vi "PreparePassReceiverRole.vi"(5 "Striker/2ndStriker":T1, 6 "Tactic index in":i32, 7 "first call":bool, 8 "error in (no error)":errorcluster, 9 "RobotRef":refnum<class "Robot.lvclass">, 10 "Game in":refnum<class "Game.lvclass">, 11 "PreparePassReceiverRole in":refnum<class "PreparePassReceiverRole.lvclass">) -> (0 "error out":errorcluster, 1 "Robot out":refnum<class "Robot.lvclass">, 2 "Game out":refnum<class "Game.lvclass">, 3 "PreparePassReceiverRole out":refnum<class "PreparePassReceiverRole.lvclass">, 4 "tactic index":i32)   [LabVIEW 2023, in "PreparePassReceiverRole.lvclass"]
uses:
  PreparePassReceiverRole.lvclass
  Game_class/Game.lvclass
  Robot_class/Robot.lvclass
  PreparePassReceiverEnum.ctl
  Role_class/Role.lvclass/Role.ctl
  PositionToReceivePassTactic_class/PositionToReceivePassTactic.lvclass/PositionToReceivePassTactic.ctl
  PositionToReceivePassTactic_class/Read States.vi
  Role_class/Read Tacticbook.vi
  Role_class/Write Tacticbook.vi
  Role_class/Write tactic_index.vi
  Tacticbook_class/Tacticbook.lvclass
  PositionToReceivePassTactic_class/PositionToReceivePassTactic.lvclass
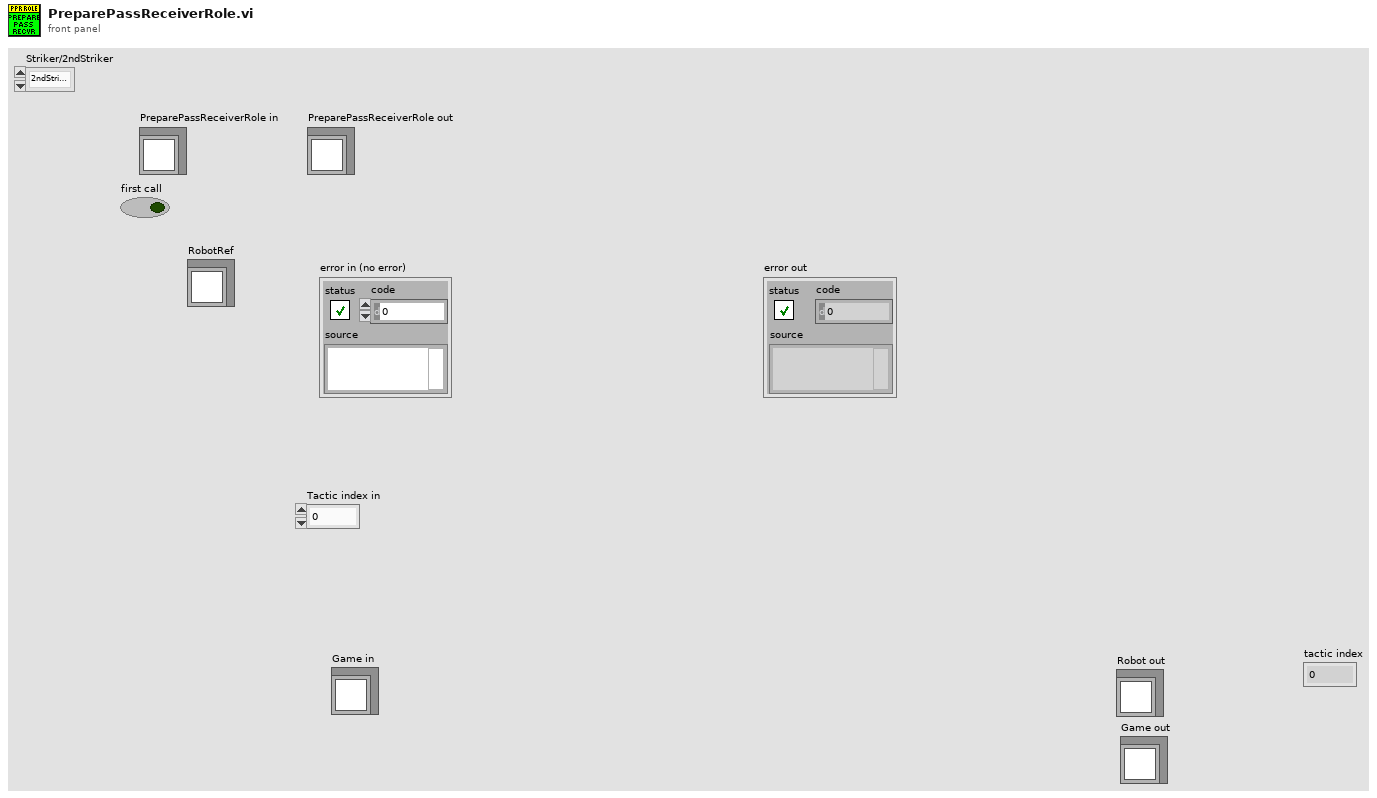
[diagram p1: front panel]
types:
  T1 = typedef "PreparePassReceiverEnum.ctl" = enum16{"2ndStrikerDPass", "2ndStriker", "Striker"}
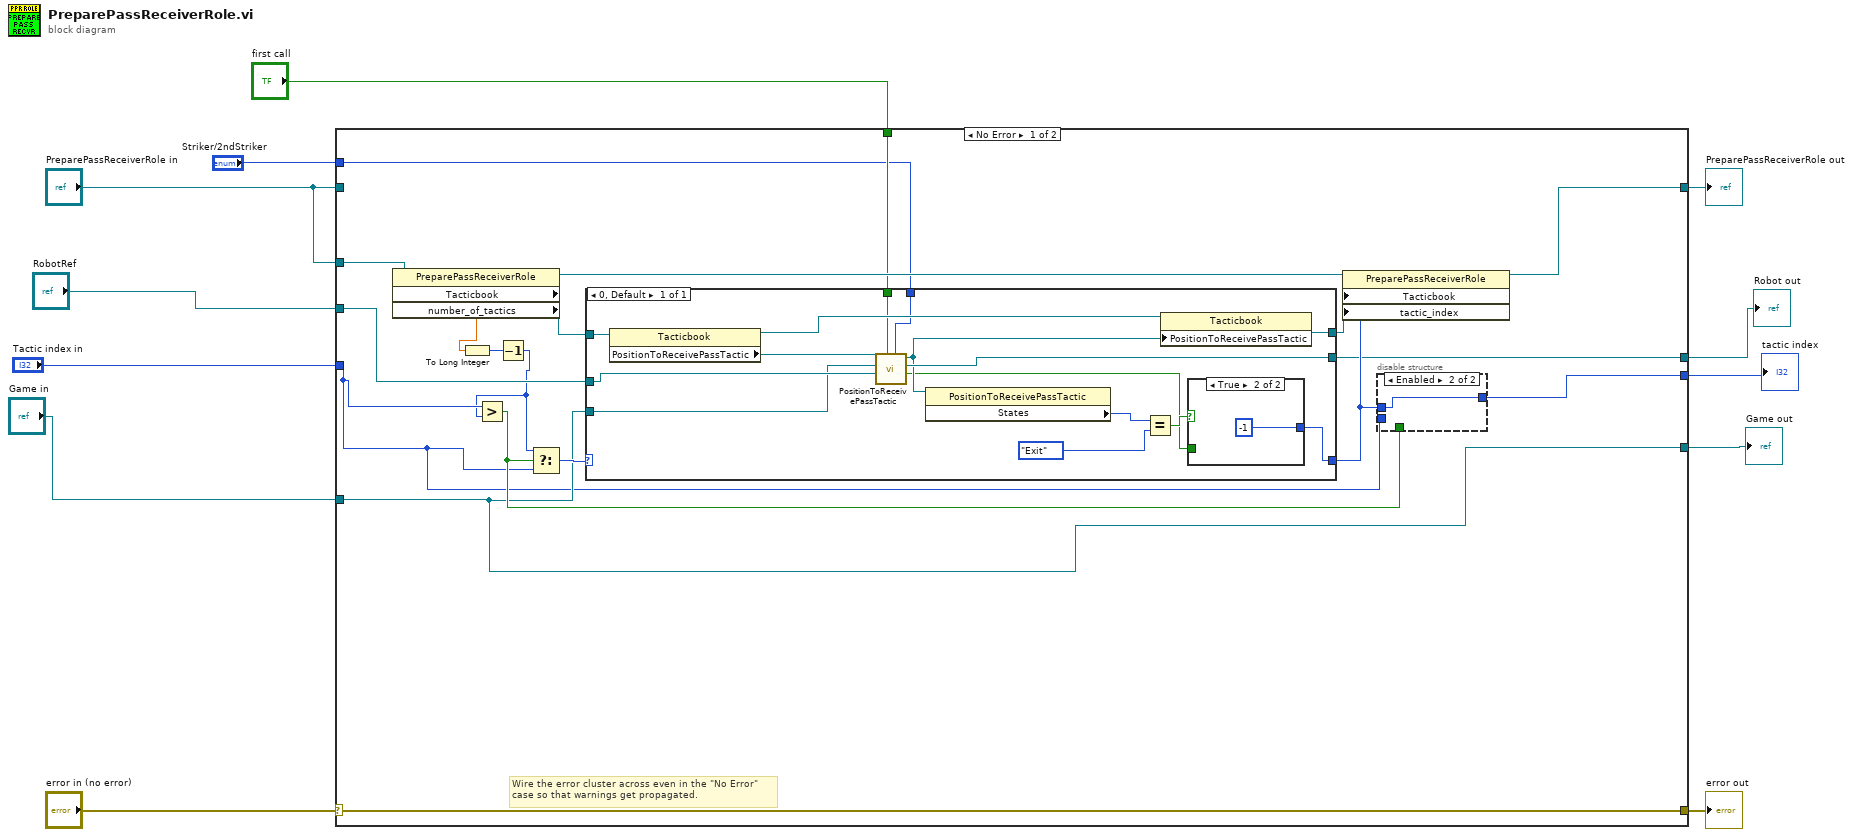
[diagram p0: block diagram]
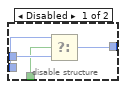
[diagram p2: hidden frame]
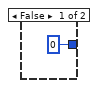
[diagram p3: hidden frame]
diagram:
  n1 = case shown="No Error" "error in (no error)" {
    selector: "error in (no error)" -> [w31 w55]
    tunnel: [w31 w55] -> w11
    tunnel: [w19 w54] -> w10
    tunnel: "PreparePassReceiverRole in" -> [_ w54]
    tunnel: "first call" -> [w24 _]
    tunnel: [w23 _] -> w8
    tunnel: [w22 _] -> w7
    tunnel: "Game in" -> [w21 _]
    tunnel: [w21 _] -> w5
    tunnel: "PreparePassReceiverRole in" -> [w20 _]
    tunnel: "Tactic index in" -> [w18 _]
    tunnel: "RobotRef" -> [w17 _]
    tunnel: "Striker/2ndStriker" -> [w16 _]
    frame No Error {
      # "Wire the error cluster across even in the \"No Error\"\ncase so that warnings get propagated."
      n2 = property class="PreparePassReceiverRole"(reference=w20) -> (reference out=w30:refnum<class "PreparePassReceiverRole.lvclass">, "Tacticbook"=w29:refnum<class "Tacticbook.lvclass">, "number_of_tactics"=w15:dbl)  [unwired: 1 in, 1 out]
      n3 = To Long Integer(number=w15) -> (32bit integer=w14:i32)
      n4 = Decrement(x=w14) -> (x-1=w13:i32)
      n5 = Greater?(x=w18, y=w13) -> (0:w25:bool)
      n6 = Select(t=w13, s=w25, f=w18) -> (s? t:f=w26:i32)
      n7 = case shown="0, Default" w26 {
        tunnel: [w42] -> w27
        tunnel: w29 -> [w51]
        tunnel: w17 -> [w46]
        tunnel: [w50] -> w23
        tunnel: [w48] -> w28
        tunnel: w21 -> [w45]
        tunnel: w24 -> [w41]
        tunnel: w16 -> [w38]
        frame 0, Default {
          n8 = property class="Tacticbook"(reference=w51) -> (reference out=w49:refnum<class "Tacticbook.lvclass">, "PositionToReceivePassTactic"=w47:refnum<class "PositionToReceivePassTactic.lvclass">)  [unwired: 1 in, 1 out]
          n9 = call "PositionToReceivePassTactic.vi"("Striker/2ndStriker"=w38, "first call"=w41, "Robot"=w46, "Game in"=w45, "PositionToReceivePassTactic in"=w47) -> ("Sucsses"=w37:bool, "Robot out"=w50:refnum<class "Robot.lvclass">, "PositionToReceivePassTactic out"=w44:refnum<class "PositionToReceivePassTactic.lvclass">)  [unwired: 3 in, 1 out]
          n10 = property class="PositionToReceivePassTactic"(reference=w44) -> ("States"=w39:enum16{"ReceivePass", "Exit"})  [unwired: 1 in, 2 out]
          n11 = Equal?(x=w39, y=enum16{"ReceivePass", "Exit"}."Exit" ("States")) -> (x = y?=w43:bool)
          n12 = property class="Tacticbook"(reference=w49, "PositionToReceivePassTactic"=w44) -> (reference out=w48:refnum<class "Tacticbook.lvclass">)  [unwired: 1 in, 1 out]
          n13 = case shown="True" w43 {
            tunnel: [0 -1] -> w42
            tunnel: w37 -> [_ _]
            frame False {
            }
            frame True {
            }
          }
        }
      }
      n14 = property class="PreparePassReceiverRole"(reference=w30, "Tacticbook"=w28, "tactic_index"=w27) -> (reference out=w19:refnum<class "PreparePassReceiverRole.lvclass">)  [unwired: 1 in, 1 out]
      n15 = disable-structure shown="Enabled" {
        disable-tunnel: w27 -> [w35 w36]
        disable-tunnel: w25 -> [w34 _]
        disable-tunnel: [w33 w36] -> w22
        disable-tunnel: w18 -> [w32 _]
        frame Disabled {
          n16 = Select(t=w32, s=w34, f=w35) -> (s? t:f=w33:i32)
        }
        frame Enabled {
        }
      }
    }
    frame Error {
    }
  }
  "error out" <- w11
  "PreparePassReceiverRole out" <- w10
  "Robot out" <- w8
  "Game out" <- w5
  "tactic index" <- w7
